vi "[Global] Coord.vi"() -> ()   [LabVIEW 2019]
panel:
  out "CoordArray":string[](array[string])
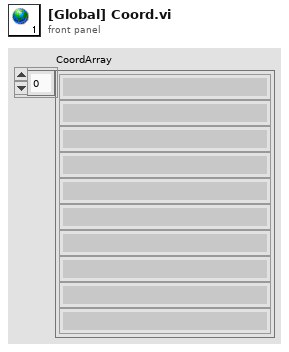
[diagram p1: front panel]
diagram:
